vi "Flatten Pixmaps - GIF__ogtk.vi"(10 "GlobalColorTable(GIF)":bool, 11 "PixelTable":u32[][][](array[colorbox])) -> (3 "Images":T1[](array[typedef]))   [LabVIEW 2020]
uses:
  <vilib>/picture/picture.llb/imagedata.ctl
panel:
  # "GIF can encode multiple images and each image can have it's own Color table, however this may enlarge the gif by up to 768 bytes/image (3 bytes/color, 256 colors).\n\nIf less than 256 colors, are present in all the images together, set \"GlobalColorTable(GIF)\" = True, so all \"Images\" will use the GIF's  Global Color table."
  # "Util.Pict.PixelTableToImage.vi\n\nConverts a sequence of PixelTables to an array of \"image data\" clusters.\n\nPlease visit http://www.OpenG.org to learn about the\nOpen Source LabVIEW software movement.\n\nNOTICE -- YOU MUST LEAVE THIS NOTICE IN PLACE.  PER THE TERMS OF THE LICENSE BELOW, YOU MAY SUBLICENSE THIS SOFTWARE \nIN ANY WAY THAT DOES NOT CONFLICT WITH THIS LICENSE.\n\n### BSD License (http://www.opensource.org/licenses/bsd-license.php) Begin ###\n \nCopyright (c) 2007, Bill Clench <bclench@yahoo.com>\n\nAll rights reserved.\n\nRedistribution and use in source and binary forms, with or without modification, are permitted provided that the following conditions are met:\n\n    * Redistributions of source code must retain the above copyright notice, this list of conditions and the following disclaimer.\n    * Redistributions in binary form must reproduce the above copyright notice, this list of conditions and the following disclaimer in the \n       documentation and/or other materials provided with the distribution.\n    * Neither the name of SciWare, James Kring, Inc., nor the names of its contributors may be used to endorse or promote products derived \n       from this software without specific prior written permission.\n\nTHIS SOFTWARE IS PROVIDED BY THE COPYRIGHT HOLDERS AND CONTRIBUTORS \"AS IS\" AND ANY EXPRESS OR IMPLIED WARRANTIES, \nINCLUDING, BUT NOT LIMITED TO, THE IMPLIED WARRANTIES OF MERCHANTABILITY AND FITNESS FOR A PARTICULAR PURPOSE ARE \nDISCLAIMED. IN NO EVENT SHALL THE COPYRIGHT OWNER OR CONTRIBUTORS BE LIABLE FOR ANY DIRECT, INDIRECT, INCIDENTAL,\n SPECIAL, EXEMPLARY, OR CONSEQUENTIAL DAMAGES (INCLUDING, BUT NOT LIMITED TO, PROCUREMENT OF SUBSTITUTE GOODS OR \nSERVICES; LOSS OF USE, DATA, OR PROFITS; OR BUSINESS INTERRUPTION) HOWEVER CAUSED AND ON ANY THEORY OF LIABILITY, \nWHETHER IN CONTRACT, STRICT LIABILITY, OR TORT (INCLUDING NEGLIGENCE OR OTHERWISE) ARISING IN ANY WAY OUT OF THE USE \nOF THIS SOFTWARE, EVEN IF ADVISED OF THE POSSIBILITY OF SUCH DAMAGE.\n\n### BSD License End ###"
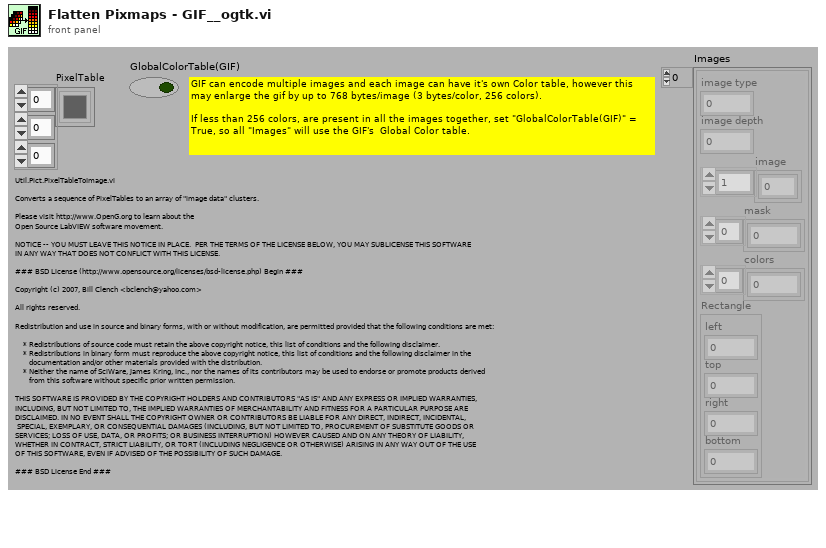
[diagram p1: front panel]
types:
  T1 = typedef "imagedata.ctl" = cluster{"image type":i32, "image depth":i32, "image":u8[], "mask":u8[], "colors":u32[], "Rectangle":cluster{"left":i16, "top":i16, "right":i16, "bottom":i16}}
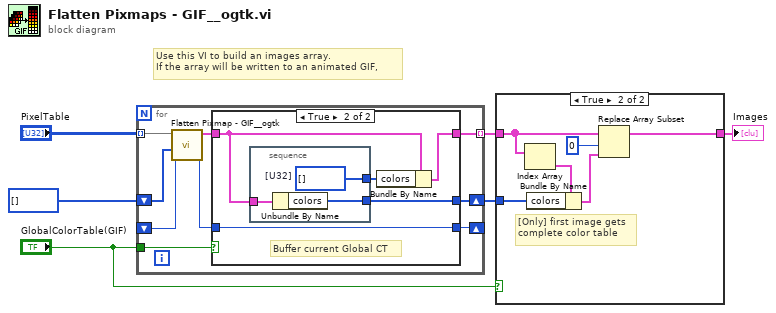
[diagram p0: block diagram]
diagram:
  # "Use this VI to build an images array.\nIf the array will be written to an animated GIF,"
  n1 = for {
    tunnel: "PixelTable" -> [w15] mode=indexing
    tunnel: [w10] -> w5 mode=indexing
    tunnel: "GlobalColorTable(GIF)" -> [w11]
    shift-right: [w12] -> w3
    shift-left: u32[] [] -> [w14]
    shift-right: [w7] -> _
    shift-left: _ -> [w9]
    n2 = call <userlib>:"Flatten Pixmap - GIF__ogtk.vi"("StartColorIndex"=w9, "ExistingColorTable"=w14, "PixelTable"=w15) -> ("EndColorIndex"=w8:i32, "image data"=w13:T1)  [unwired: 7 in]
    n3 = case shown="True" w11 {
      tunnel: w13 -> [w16 w20]
      tunnel: [_ w21] -> w12
      tunnel: [w16 w18] -> w10
      tunnel: w8 -> [_ w17]
      tunnel: [_ w17] -> w7
      frame False {
        # "Each image starts with\nempty color-table, so\nit will construct its own."
      }
      frame True {
        # "Buffer current Global CT"
        n4 = stacked-sequence {
          tunnel: [w24] -> w21
          tunnel: w20 -> [w23]
          tunnel: [w22] -> w19
          frame #0 {
            w22 = u32[] []  # [U32]
            n5 = Unbundle By Name(w23) -> ("colors"=w24:u32[])
          }
        }
        n6 = Bundle By Name(cluster=w20, "colors"=w19) -> (w18:T1)
      }
    }
  }
  n7 = case shown="True" "GlobalColorTable(GIF)" {
    tunnel: w5 -> [w25 w31]
    tunnel: [w25 w30] -> w4
    tunnel: w3 -> [_ w28]
    frame False {
    }
    frame True {
      # "[Only] first image gets\ncomplete color table"
      n8 = Index Array(array=w31) -> (element=w29:T1)  [unwired: 1 in]
      n9 = Bundle By Name(cluster=w29, "colors"=w28) -> (w27:T1)
      n10 = Replace Array Subset "Replace Array Subset"(array=w31, new element=w27, index=0) -> (w30:T1[])
    }
  }
  "Images" <- w4
